vi "Insert.vi"(6 "Time Stamp":timestamp, 7 "backup storage folder":path, 8 "error in":errorcluster, 9 "Data":variant, 10 "Paths (string or array of strings)":variant, 11 "Data.PG in":refnum<class "Data.PG.lvclass">) -> (0 "error out":errorcluster, 1 "Wrote to DB?":bool, 3 "Data.PG out":refnum<class "Data.PG.lvclass">)   [LabVIEW 2020, in "Data.PG.lvclass"]
uses:
  Data.PG.lvclass
  Data/Typedefs/Operation--enum.ctl
  <vilib>/Utility/error.llb/DialogType.ctl
  Data.PG.lvclass/Data.PG.ctl
  <vilib>/JDP Science/PostgreSQL Library/Result/PQ Result.lvclass/PQ Result.ctl
  <vilib>/JDP Science/PostgreSQL Library/Connection/Execute Command (No results).vi
  <vilib>/JDP Science/PostgreSQL Library/Result/Clear.vi
  <vilib>/JDP Science/PostgreSQL Library/Connection/Execute Command (Result).vi
  <vilib>/JDP Science/PostgreSQL Library/Connection/Execute (Return first result with rows).vi
  <vilib>/JDP Science/PostgreSQL Library/Connection/Single Command with parameters.vi
  <vilib>/JDP Science/PostgreSQL Library/Connection/PQ Connection.lvclass
  Data/Data.lvclass
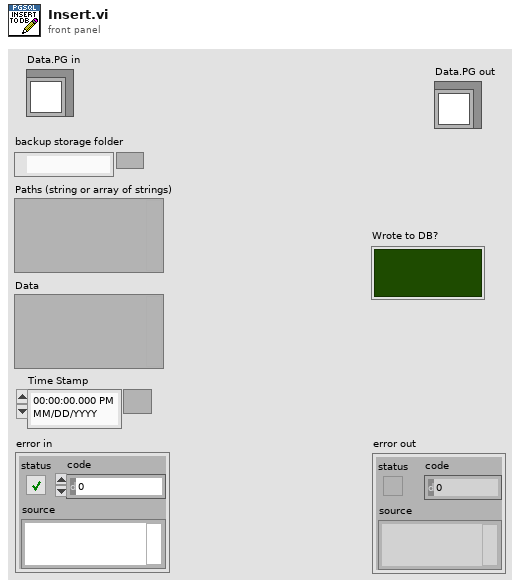
[diagram p1: front panel]
types:
  T1 = typedef "Data.lvclass/Operation--enum.ctl" = enum16{"Read", "Write", "Write + Append"}
  T2 = typedef "DialogType.ctl" = u16
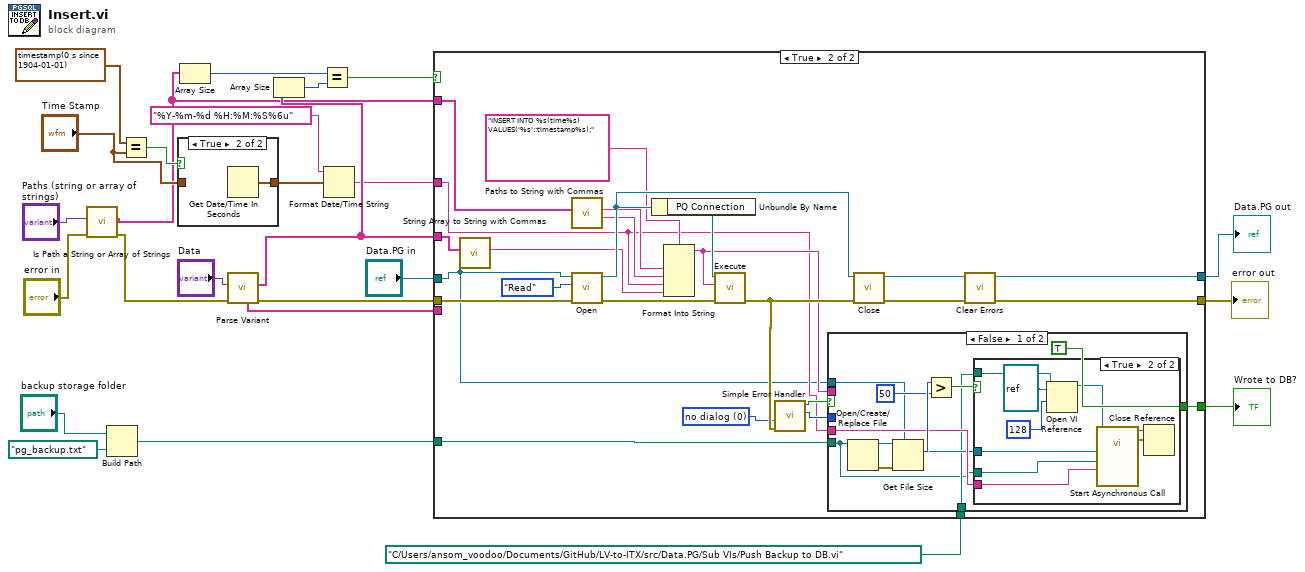
[diagram p0: block diagram]
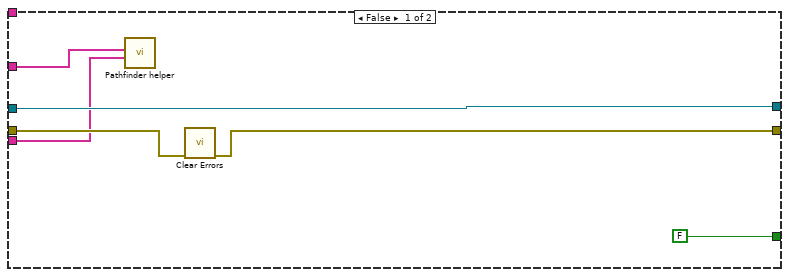
[diagram p2: hidden frame]
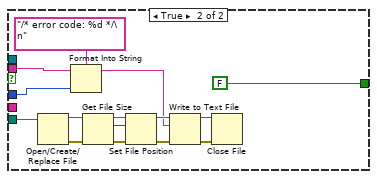
[diagram p4: hidden frame]
diagram:
  n1 = call "Is Path a String or Array of Strings.vi"("error in"="error in", "Paths?"="Paths (string or array of strings)") -> ("error out"=w7:errorcluster, "Paths."=w9:string[])  [unwired: 8 in]
  n2 = Build Path(base path="backup storage folder", name or relative path=path "pg_backup.txt") -> (appended path=w3:path)
  n3 = Equal?(x=timestamp(0 s since 1904-01-01), y="Time Stamp") -> (x = y?=w22:bool)
  n4 = case shown="True" w22 {
    tunnel: [w26 w27] -> w23
    tunnel: "Time Stamp" -> [w26 _]
    frame False {
    }
    frame True {
      n5 = Get Date/Time In Seconds() -> (seconds since 1Jan1904=w27:timestamp)
    }
  }
  n6 = Array Size(array=w9) -> (size(s)=w19:i32)
  n7 = call "Parse Variant.vi"("error in"=w7, "variant"="Data") -> ("error out"=w14:errorcluster, "Strings"=w16:string[], "Types (strings)"=w6:string[])  [unwired: 5 in, 2 out]
  n8 = Array Size(array=w16) -> (size(s)=w18:i32)
  n9 = Equal?(x=w19, y=w18) -> (x = y?=w17:bool)
  n10 = Format Date/Time String(time format string (%c)="%Y-%m-%d %H:%M:%S%6u", seconds (now)=w23) -> (date/time string=w13:string)  [unwired: 1 in]
  n11 = case shown="True" w17 {
    tunnel: w16 -> [w30 w57]
    tunnel: w9 -> [_ w56]
    tunnel: [w31 w41] -> w15
    tunnel: w14 -> [w32 w53]
    tunnel: w13 -> [_ w36]
    tunnel: "Data.PG in" -> [w33 w35]
    tunnel: [w33 w48] -> w11
    tunnel: w6 -> [w29 _]
    tunnel: w3 -> [_ w38]
    tunnel: [FALSE w37] -> w2
    tunnel: path "C:/Users/ansom_voodoo/Documents/GitHub/LV-to-ITX/src/Data.PG/Sub VIs/Push Backup to DB.vi" ("vi path") -> [_ w34]
    frame False {
      n12 = call "Pathfinder helper.vi"("Types (string)"=w29, "Data"=w30) -> ()  [unwired: 10 in]
      n13 = call <vilib>:"Clear Errors.vi"("error in (no error)"=w32) -> ("error out"=w31:errorcluster)  [unwired: 5 in, 1 out]
    }
    frame True {
      w39 = T2 0 items=["no dialog", "OK message", "continue or stop message", "OK message + warnings", "continue/stop + warnings"] ("type of dialog (OK msg:1)")
      n14 = call "String Array to String with Commas.vi"("Array"=w57) -> ("String"=w50:string)  [unwired: 10 in]
      n15 = call "Paths to String with Commas.vi"("Array"=w56) -> ("Columns"=w51:string, "Table"=w52:string)  [unwired: 9 in]
      n16 = call-dynamic "Open.vi"("error in (no error)"=w53, "Operation"=Operation--enum."Read", "Data.PG in"=w35) -> ("error out"=w47:errorcluster, "Data.PG out"=w54:refnum<class "Data.PG.lvclass">)  [unwired: 7 in]
      n17 = Unbundle By Name(w54) -> ("PQ Connection"=w49:refnum<class "PQ Connection.lvclass">)
      n18 = Format Into String(format string="INSERT INTO %s(time%s) VALUES('%s'::timestamp%s);", w52, w51, w36, w50) -> (resulting string=w40:string)  [unwired: 2 in, 1 out]
      n19 = call-poly <vilib>:"Execute.vi"("error in (no error)"=w47, "SQL"=w40, "PQ Connection in"=w49) -> ("error out"=w46:errorcluster)  [unwired: 7 in, 1 out]
      n20 = call <vilib>:"Simple Error Handler.vi"("type of dialog (OK msg:1)"=w39, "error in (no error)"=w46) -> ("error?"=w45:bool, "code out"=w43:i32)  [unwired: 3 in, 3 out]
      n21 = case shown="False" w45 {
        tunnel: w40 -> [_ w89]
        tunnel: w43 -> [_ w90]
        tunnel: w38 -> [w58 w88]
        tunnel: [TRUE FALSE] -> w37
        tunnel: w36 -> [w61 _]
        tunnel: w35 -> [w60 _]
        tunnel: w34 -> [w59 _]
        frame False {
          n22 = Open/Create/Replace File(file path (use dialog)=w58) -> (refnum out=w65:refnum<file>, error out=w66:errorcluster)  [unwired: 5 in, 1 out]
          n23 = Get File Size(file=w65, error in=w66) -> (size (in bytes)=w64:i64)  [unwired: 2 out]
          n24 = Greater?(x=w64, y=i64 50) -> (0:w62:bool)
          n25 = case shown="True" w62 {
            tunnel: w61 -> [_ w70]
            tunnel: w60 -> [_ w72]
            tunnel: w59 -> [_ w76]
            tunnel: w58 -> [_ w71]
            frame False {
            }
            frame True {
              n26 = Open VI Reference(type specifier VI Refnum (for type only)=refnum<vi> refnum, vi path=w76, options=128) -> (vi reference=w74:refnum<vi>)  [unwired: 3 in, 1 out]
              n27 = call-by-ref "Start Asynchronous Call"(reference=w74, "timestamp string"=w70, "Path to backup file"=w71, "Data.PG in"=w72) -> (reference out=w68:refnum<vi>, error out=w69:errorcluster)  [unwired: 10 in]
              n28 = Close Reference(reference=w68, error in (no error)=w69) -> ()  [unwired: 1 out]
            }
          }
        }
        frame True {
          n29 = Open/Create/Replace File(file path (use dialog)=w88) -> (refnum out=w86:refnum<file>, error out=w87:errorcluster)  [unwired: 5 in, 1 out]
          n30 = Format Into String(format string="/* error code: %d */\n", initial string=w89, w90) -> (resulting string=w80:string)  [unwired: 1 in, 1 out]
          n31 = Get File Size(file=w86, error in=w87) -> (refnum out=w83:refnum<file>, size (in bytes)=w84:i64, 0:w85:errorcluster)
          n32 = Set File Position(offset (in bytes) (0)=w84, refnum=w83, error in=w85) -> (refnum out=w81:refnum<file>, error out=w82:errorcluster)  [unwired: 1 in]
          n33 = Write to Text File(file (use dialog)=w81, text=w80, error in=w82) -> (refnum out=w78:refnum<file>, error out=w79:errorcluster)  [unwired: 1 in, 1 out]
          n34 = Close File(refnum=w78, error in=w79) -> ()  [unwired: 2 out]
        }
      }
      n35 = call-dynamic "Close.vi"("error in (no error)"=w46, "Data.PG in"=w54) -> ("error out"=w42:errorcluster, "Data.PG out"=w48:refnum<class "Data.PG.lvclass">)  [unwired: 8 in]
      n36 = call <vilib>:"Clear Errors.vi"("error in (no error)"=w42) -> ("error out"=w41:errorcluster)  [unwired: 5 in, 1 out]
    }
  }
  "error out" <- w15
  "Data.PG out" <- w11
  "Wrote to DB?" <- w2
